vi "DLS Profile.vi"(0 "GEA2 Reference In":refnum<k24>, 1 "Shift To":enum16{"Spin", "Agitate"}(ring), 2 "Input Bit":T3, 5 "GEA Inputs":T4={"Source"=228, "Destination"=35} {"Destination" format="%.0x"; "Source" format="%.0x"}, 7 "Standalone?":bool, 11 "Error In":errorcluster, 12 "Action":enum16{"Lock", "Unlock"}(ring), 13 "Co-efficient Data":T2) -> (4 "GEA2 Reference Out":refnum<k24>, 6 "Calc_Dry Load Size":dbl, 8 "Expected_Dry Load Size":dbl, 10 "Report Text":string, 14 "Pass/Fail":bool, 15 "Error Out":errorcluster)   [LabVIEW 2016, in "2015 VA Washer.lvlib"]
uses:
  Projects/2015 VA Washer.lvlib
  C:/Automation/DLLs/PC Dot Net/GeaCommunication.dll
  Common/LabVIEW GEA2 Toolkit/LabVIEW_GEA2_Toolkit.lvlibp/type defs/Source_Destination.ctl
  Control/DLS ERD Data.ctl
  Valew Common/type defs/Drive Cycle Engine Request State.ctl
  Common/LabVIEW GEA2 Toolkit/LabVIEW_GEA2_Toolkit.lvlibp/type defs/ERD Read Data In.ctl
  Common/LabVIEW GEA2 Toolkit/LabVIEW_GEA2_Toolkit.lvlibp/type defs/Data Type.ctl
  Common/LabVIEW GEA2 Toolkit/LabVIEW_GEA2_Toolkit.lvlibp
panel:
  out "R1_R2_R3_DLS (Q5)":dbl
  out "R1_R2 Avg_DLS (Q5)":dbl
  out "R3_DLS ERD Data":T1
  out "R3_Result Q5 Tranformation":dbl
  out "R2_DLS ERD Data":T1
  out "R2_Result Q5 Tranformation":dbl
  out "R1_Result Q5 Tranformation":dbl
  out "R1_DLS ERD Data":T1
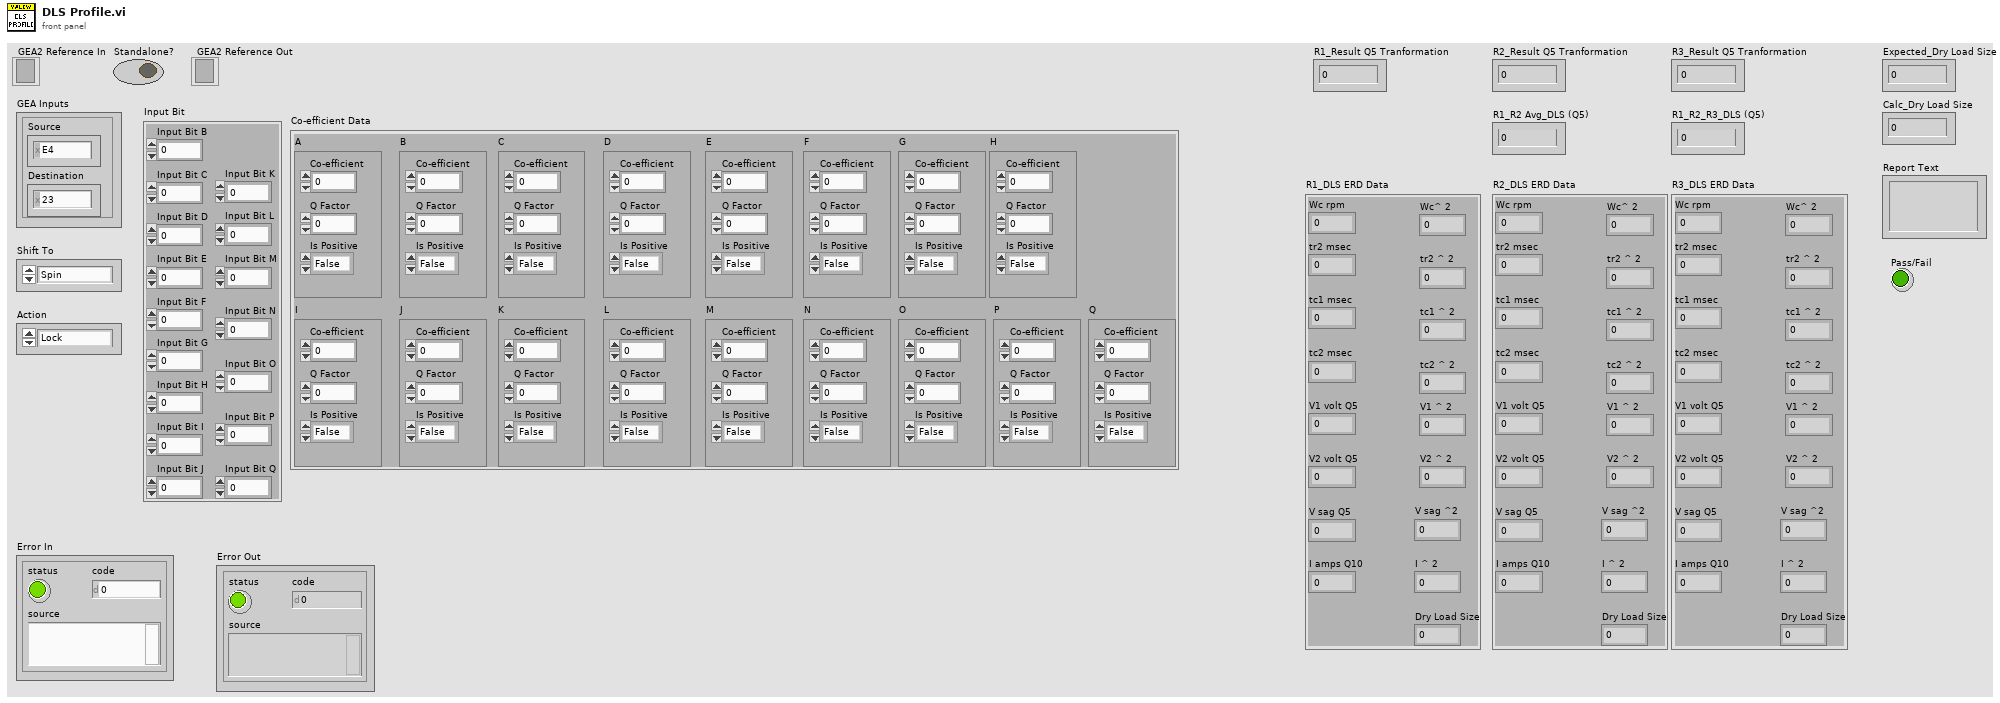
[diagram p1: front panel]
types:
  T1 = typedef "2015 VA Washer.lvlib/DLS ERD Data.ctl" = cluster{"Wc rpm":dbl, "tr2 msec":dbl, "tc1 msec":dbl, "tc2 msec":dbl, "V1 volt Q5":dbl, "V2 volt Q5":dbl, "I amps Q10":dbl, "Wc^ 2":dbl, "tr2 ^ 2":dbl, "tc1 ^ 2":dbl, "tc2 ^ 2":dbl, "V1 ^ 2":dbl, "V2 ^ 2":dbl, "I ^ 2":dbl, "V sag Q5":dbl, "V sag ^2":dbl, "Dry Load Size":dbl}
  T2 = cluster{"A":cluster{"Co-efficient":dbl, "Q Factor":dbl, "Is Positive":enum16{"False", "True"}}, "B":cluster{"Co-efficient":dbl, "Q Factor":dbl, "Is Positive":enum16{"False", "True"}}, "C":cluster{"Co-efficient":dbl, "Q Factor":dbl, "Is Positive":enum16{"False", "True"}}, "D":cluster{"Co-efficient":dbl, "Q Factor":dbl, "Is Positive":enum16{"False", "True"}}, "E":cluster{"Co-efficient":dbl, "Q Factor":dbl, "Is Positive":enum16{"False", "True"}}, "F":cluster{"Co-efficient":dbl, "Q Factor":dbl, "Is Positive":enum16{"False", "True"}}, "G":cluster{"Co-efficient":dbl, "Q Factor":dbl, "Is Positive":enum16{"False", "True"}}, "H":cluster{"Co-efficient":dbl, "Q Factor":dbl, "Is Positive":enum16{"False", "True"}}, "I":cluster{"Co-efficient":dbl, "Q Factor":dbl, "Is Positive":enum16{"False", "True"}}, "J":cluster{"Co-efficient":dbl, "Q Factor":dbl, "Is Positive":enum16{"False", "True"}}, "K":cluster{"Co-efficient":dbl, "Q Factor":dbl, "Is Positive":enum16{"False", "True"}}, "L":cluster{"Co-efficient":dbl, "Q Factor":dbl, "Is Positive":enum16{"False", "True"}}, "M":cluster{"Co-efficient":dbl, "Q Factor":dbl, "Is Positive":enum16{"False", "True"}}, "N":cluster{"Co-efficient":dbl, "Q Factor":dbl, "Is Positive":enum16{"False", "True"}}, "O":cluster{"Co-efficient":dbl, "Q Factor":dbl, "Is Positive":enum16{"False", "True"}}, "P":cluster{"Co-efficient":dbl, "Q Factor":dbl, "Is Positive":enum16{"False", "True"}}, "Q":cluster{"Co-efficient":dbl, "Q Factor":dbl, "Is Positive":enum16{"False", "True"}}}
  T3 = cluster{"Input Bit B":dbl, "Input Bit C":dbl, "Input Bit D":dbl, "Input Bit E":dbl, "Input Bit F":dbl, "Input Bit G":dbl, "Input Bit H":dbl, "Input Bit I":dbl, "Input Bit J":dbl, "Input Bit K":dbl, "Input Bit L":dbl, "Input Bit M":dbl, "Input Bit N":dbl, "Input Bit O":dbl, "Input Bit P":dbl, "Input Bit Q":dbl}
  T4 = typedef "LabVIEW_GEA2_Toolkit.lvlibp/Source_Destination.ctl" = cluster{"Source":u8, "Destination":u8}
  T5 = enum16{"EQ (==)", "NE (!=)", "GT (>)", "LT (<)", "GE (>=)", "LE (<=)", "GTLT(> <)", "GELE (>= <=)", "GELT (>= <)", "GTLE (> <=)", "LTGT (< >)", "LEGE (<= >=)", "LEGT (<= >)", "LTGE (< >=)", "No Comparison"}
  T6 = typedef "LabVIEW_GEA2_Toolkit.lvlibp/ERD Read Data In.ctl" = cluster{"ERD Number":u16, "Data Type":T7}
  T7 = typedef "LabVIEW_GEA2_Toolkit.lvlibp/Data Type.ctl" = enum16{"string", "boolean", "uint8_t", "uint16_t", "uint32_t", "uint64_t", "int8_t", "int16_t", "int32_t", "int64_t"}
  T8 = typedef "2015 VA Washer.lvlib/Drive Cycle Engine Request State.ctl" = enum16{"Start", "Stop", "Pause", "Resume", "Select"}
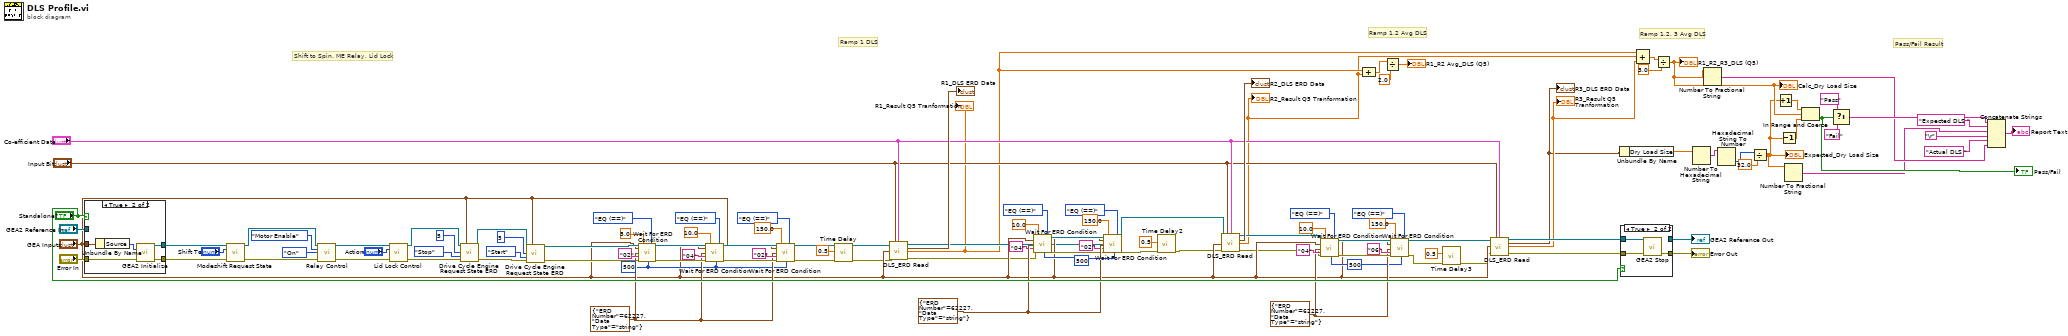
[diagram p0: block diagram]
diagram:
  w47 = u32 500 ("Loop Rate (ms)")
  w50 = T6 {"ERD Number"=62227, "Data Type"=enum."string"} ("ERD Read Data")
  w67 = u32 500 ("Loop Rate (ms)")
  w64 = T6 {"ERD Number"=62227, "Data Type"=enum."string"} ("ERD Read Data")
  w70 = u32 500 ("Loop Rate (ms)")
  w73 = T6 {"ERD Number"=62227, "Data Type"=enum."string"} ("ERD Read Data")
  # "Shift to Spin, ME Relay, Lid Lock"
  # "Ramp 1 DLS"
  # "Ramp 1,2 Avg DLS"
  # "Ramp 1,2, 3 Avg DLS"
  # "Pass/Fail Result"
  n1 = case shown="True" "Standalone?" {
    tunnel: "GEA2 Reference In" -> [w112 _]
    tunnel: [w112 w117] -> w96
    tunnel: "Error In" -> [w111 w116]
    tunnel: [w111 w115] -> w94
    tunnel: "GEA Inputs" -> [_ w114]
    frame False {
    }
    frame True {
      n2 = Unbundle By Name(w114) -> ("Source"=w113:u8)
      n3 = call "GEA2 Initialize.vi"("Source Address"=w113, "error in"=w116) -> ("GEA2 Reference Out"=w117:refnum<k24>, "error out"=w115:errorcluster)  [unwired: 11 in, 1 out]
    }
  }
  n4 = call "Modeshift Request State.vi"("GEA2 Reference In"=w96, "Shift To"="Shift To", "Error In"=w94) -> ("GEA2 Reference Out"=w95:refnum<k24>, "Error Out"=w93:errorcluster)  [unwired: 9 in, 2 out]
  n5 = call "Relay Control.vi"("GEA2 Reference In"=w95, "Relay"=enum16{"Motor Enable", "Valve", "Both"}."Motor Enable", "State"=enum16{"On", "Off"}."On", "Error In"=w93) -> ("GEA2 Reference Out"=w103:refnum<k24>, "Error Out"=w101:errorcluster)  [unwired: 8 in, 2 out]
  n6 = call "Lid Lock Control.vi"("GEA2 Reference In"=w103, "Action"="Action", "Error In"=w101) -> ("GEA2 Reference Out"=w102:refnum<k24>, "Error Out"=w100:errorcluster)  [unwired: 9 in, 2 out]
  n7 = call "Drive Cycle Engine Request State ERD.vi"("GEA2 Reference In"=w102, "GEA Inputs"="GEA Inputs", "Cycle ID"=u8 5, "Drive Cycle Engine Request State"=Drive_Cycle_Engine_Request_State."Stop", "Error In"=w100) -> ("GEA2 Reference Out"=w91:refnum<k24>, "Error Out"=w90:errorcluster)  [unwired: 9 in]
  n8 = call "Drive Cycle Engine Request State ERD.vi"("GEA2 Reference In"=w91, "GEA Inputs"="GEA Inputs", "Cycle ID"=u8 5, "Drive Cycle Engine Request State"=Drive_Cycle_Engine_Request_State."Start", "Error In"=w90) -> ("GEA2 Reference Out"=w84:refnum<k24>, "Error Out"=w85:errorcluster)  [unwired: 9 in]
  n9 = call "Wait For ERD Condition.vi"("GEA2 Reference In"=w84, "GEA Inputs"="GEA Inputs", "ERD Read Data"=w73, "Expected Low"="02", "Error In"=w85, "Timeout (s)"=5.0, "Loop Rate (ms)"=w70, "Comparison"=T5."EQ (==)") -> ("GEA2 Reference Out"=w81:refnum<k24>, "Error Out"=w80:errorcluster)  [unwired: 7 in, 3 out]
  n10 = call "Wait For ERD Condition.vi"("GEA2 Reference In"=w81, "GEA Inputs"="GEA Inputs", "ERD Read Data"=w73, "Expected Low"="04", "Error In"=w80, "Timeout (s)"=10.0, "Loop Rate (ms)"=w70, "Comparison"=T5."EQ (==)") -> ("GEA2 Reference Out"=w76:refnum<k24>, "Error Out"=w75:errorcluster)  [unwired: 7 in, 3 out]
  n11 = call "Wait For ERD Condition.vi"("GEA2 Reference In"=w76, "GEA Inputs"="GEA Inputs", "ERD Read Data"=w73, "Expected Low"="02", "Error In"=w75, "Timeout (s)"=150.0, "Loop Rate (ms)"=w70, "Comparison"=T5."EQ (==)") -> ("GEA2 Reference Out"=w69:refnum<k24>, "Error Out"=w6:errorcluster)  [unwired: 7 in, 3 out]
  n12 = call "Time Delay"("error in (no error)"=w6, "Delay Time (s)"=0.5) -> ("error out"=w5:errorcluster)  [unwired: 9 in]
  n13 = call "DLS_ERD Read.vi"("GEA2 Reference In"=w69, "Input Bit"="Input Bit", "Co-efficient Data"="Co-efficient Data", "GEA Inputs"="GEA Inputs", "Error In"=w5) -> ("GEA2 Reference Out"=w19:refnum<k24>, "DLS ERD Data"=→"R1_DLS ERD Data":T1, "Result Q5 Tranformation"=w11:dbl, "Error Out"=w18:errorcluster)  [unwired: 7 in]
  "R1_Result Q5 Tranformation" <- w11
  n14 = call "Wait For ERD Condition.vi"("GEA2 Reference In"=w19, "GEA Inputs"="GEA Inputs", "ERD Read Data"=w64, "Expected Low"="04", "Error In"=w18, "Timeout (s)"=10.0, "Loop Rate (ms)"=w67, "Comparison"=T5."EQ (==)") -> ("GEA2 Reference Out"=w61:refnum<k24>, "Error Out"=w62:errorcluster)  [unwired: 7 in, 3 out]
  n15 = call "Wait For ERD Condition.vi"("GEA2 Reference In"=w61, "GEA Inputs"="GEA Inputs", "ERD Read Data"=w64, "Expected Low"="02", "Error In"=w62, "Timeout (s)"=150.0, "Loop Rate (ms)"=w67, "Comparison"=T5."EQ (==)") -> ("GEA2 Reference Out"=w68:refnum<k24>, "Error Out"=w4:errorcluster)  [unwired: 7 in, 3 out]
  n16 = call "Time Delay2"("error in (no error)"=w4, "Delay Time (s)"=0.5) -> ("error out"=w3:errorcluster)  [unwired: 9 in]
  n17 = call "DLS_ERD Read.vi"("GEA2 Reference In"=w68, "Input Bit"="Input Bit", "Co-efficient Data"="Co-efficient Data", "GEA Inputs"="GEA Inputs", "Error In"=w3) -> ("GEA2 Reference Out"=w17:refnum<k24>, "DLS ERD Data"=→"R2_DLS ERD Data":T1, "Result Q5 Tranformation"=w10:dbl, "Error Out"=w16:errorcluster)  [unwired: 7 in]
  "R2_Result Q5 Tranformation" <- w10
  n18 = call "Wait For ERD Condition.vi"("GEA2 Reference In"=w17, "GEA Inputs"="GEA Inputs", "ERD Read Data"=w50, "Expected Low"="04", "Error In"=w16, "Timeout (s)"=10.0, "Loop Rate (ms)"=w47, "Comparison"=T5."EQ (==)") -> ("GEA2 Reference Out"=w53:refnum<k24>, "Error Out"=w52:errorcluster)  [unwired: 7 in, 3 out]
  n19 = Compound Arithmetic op=ADD(w11, w10) -> (w40:dbl)
  n20 = Divide(x=w40, y=2.0) -> (x/y=→"R1_R2 Avg_DLS (Q5)":dbl)
  n21 = call "Wait For ERD Condition.vi"("GEA2 Reference In"=w53, "GEA Inputs"="GEA Inputs", "ERD Read Data"=w50, "Expected Low"="06", "Error In"=w52, "Timeout (s)"=150.0, "Loop Rate (ms)"=w47, "Comparison"=T5."EQ (==)") -> ("GEA2 Reference Out"=w46:refnum<k24>, "Error Out"=w2:errorcluster)  [unwired: 7 in, 3 out]
  n22 = call "Time Delay3"("error in (no error)"=w2, "Delay Time (s)"=0.5) -> ("error out"=w1:errorcluster)  [unwired: 9 in]
  n23 = call "DLS_ERD Read.vi"("GEA2 Reference In"=w46, "Input Bit"="Input Bit", "Co-efficient Data"="Co-efficient Data", "GEA Inputs"="GEA Inputs", "Error In"=w1) -> ("GEA2 Reference Out"=w42:refnum<k24>, "DLS ERD Data"=w34:T1, "Result Q5 Tranformation"=w35:dbl, "Error Out"=w41:errorcluster)  [unwired: 7 in]
  "R3_DLS ERD Data" <- w34
  "R3_Result Q5 Tranformation" <- w35
  n24 = Unbundle By Name(w34) -> ("Dry Load Size"=w31:dbl)
  n25 = case shown="True" "Standalone?" {
    tunnel: [w118 w122] -> w108
    tunnel: w41 -> [w118 w121]
    tunnel: w42 -> [w119 w120]
    tunnel: [w119 _] -> w105
    frame False {
    }
    frame True {
      n26 = call "GEA2 Stop.vi"("GEA2 Reference In"=w120, "Error In"=w121) -> ("Error Out"=w122:errorcluster)  [unwired: 13 in]
    }
  }
  "GEA2 Reference Out" <- w105
  "Error Out" <- w108
  n27 = Compound Arithmetic op=ADD(w11, w10, w35) -> (w38:dbl)
  n28 = Divide(x=w38, y=3.0) -> (x/y=w15:dbl)
  "R1_R2_R3_DLS (Q5)" <- w15
  "Calc_Dry Load Size" <- w15
  n29 = Number To Hexadecimal String(2:w31) -> (0:w24:string)  [unwired: 1 in]
  n30 = Number To Fractional String(number=w15) -> (F-format string=w14:string)  [unwired: 3 in]
  n31 = Hexadecimal String To Number(string=w24) -> (number=w33:u32)  [unwired: 2 in, 1 out]
  n32 = Divide(x=w33, y=32.0) -> (x/y=w13:dbl)
  "Expected_Dry Load Size" <- w13
  n33 = Increment(x=w13) -> (x+1=w29:dbl)
  n34 = Decrement(x=w13) -> (x-1=w30:dbl)
  n35 = Number To Fractional String(number=w13) -> (F-format string=w12:string)  [unwired: 3 in]
  n36 = In Range and Coerce(upper limit=w29, x=w15, lower limit=w30) -> (In Range?=w28:bool)  [unwired: 1 out]
  "Pass/Fail" <- w28
  n37 = Select(t="Pass", s=w28, f="Fail") -> (s? t:f=w20:string)
  n38 = Concatenate Strings(w20, "Expected DLS " ("string"), w12, "\r", "Actual DLS " ("string"), w14) -> (→"Report Text":string)
